vi "Set Constant Variables.vi"   [LabVIEW 2012]
uses:
  Robot Global Data.vi
types:
  T1 = cluster{"FVoltConst":dbl, "FVoltConst":dbl, "FVoltConst":dbl}
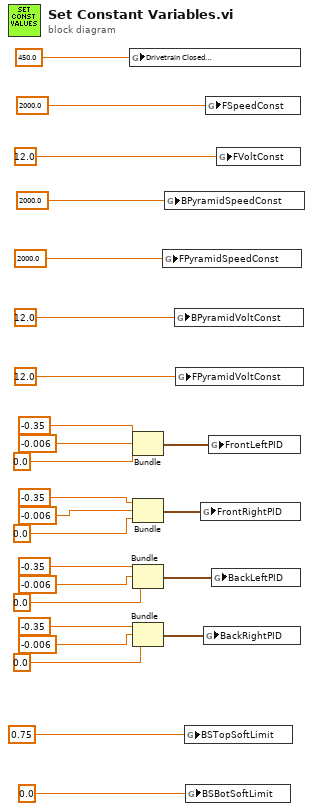
[diagram p0: block diagram]
diagram:
  n1 = global write "Robot Global Data.vi" "Drivetrain Closed\nLoop Max"(450.0 ("Drivetrain Closed\nLoop Max")) -> ()
  n2 = Bundle("FVoltConst"=-0.35, "FVoltConst"=-0.006, "FVoltConst"=0.0) -> (w20:T1)  [unwired: 1 in]
  n3 = Bundle("FVoltConst"=-0.35, "FVoltConst"=-0.006, "FVoltConst"=0.0) -> (w18:T1)  [unwired: 1 in]
  n4 = Bundle("FVoltConst"=-0.35, "FVoltConst"=-0.006, "FVoltConst"=0.0) -> (w19:T1)  [unwired: 1 in]
  n5 = Bundle("FVoltConst"=-0.35, "FVoltConst"=-0.006, "FVoltConst"=0.0) -> (w17:T1)  [unwired: 1 in]
  n6 = global write "Robot Global Data.vi" "FPyramidSpeedConst"(2000.0 ("FSpeedConst")) -> ()
  n7 = global write "Robot Global Data.vi" "BPyramidSpeedConst"(2000.0 ("FSpeedConst")) -> ()
  n8 = global write "Robot Global Data.vi" "BPyramidVoltConst"(12.0 ("FVoltConst")) -> ()
  n9 = global write "Robot Global Data.vi" "FPyramidVoltConst"(12.0 ("FVoltConst")) -> ()
  n10 = global write "Robot Global Data.vi" "BSTopSoftLimit"(0.75 ("FVoltConst")) -> ()
  n11 = global write "Robot Global Data.vi" "BSBotSoftLimit"(0.0 ("FVoltConst")) -> ()
  n12 = global write "Robot Global Data.vi" "FrontRightPID"(w18) -> ()
  n13 = global write "Robot Global Data.vi" "BackRightPID"(w17) -> ()
  n14 = global write "Robot Global Data.vi" "FSpeedConst"(2000.0 ("FSpeedConst")) -> ()
  n15 = global write "Robot Global Data.vi" "FrontLeftPID"(w20) -> ()
  n16 = global write "Robot Global Data.vi" "BackLeftPID"(w19) -> ()
  n17 = global write "Robot Global Data.vi" "FVoltConst"(12.0 ("FVoltConst")) -> ()
